vi "Registration Map Usage.vi"() -> ()   [LabVIEW 2023]
doc: "This VI demonstrates how to use the set and map data types to create a registration map with high performance."
uses:
  Do Cleaning Action.ctl
panel:
  in  "Hotel To Check":string(combo)="Four Seasons"
  in  "Stop":bool
  in  "Hotel 4":string(combo)="Four Seasons"
  in  "Unregister 4":bool
  in  "Register 4":bool
  out "Guest 4":string="Darshan"
  in  "Hotel 3":string(combo)="Four Seasons"
  in  "Unregister 3":bool
  in  "Register 3":bool
  out "Guest 3":string="Carmichael"
  in  "Hotel 2":string(combo)="Four Seasons"
  in  "Unregister 2":bool
  in  "Register 2":bool
  out "Guest 2":string="Bernice"
  in  "Hotel 1":string(combo)="Four Seasons"
  out "Event Log":string
  in  "Check":bool
  in  "Unregister 1":bool
  in  "Register 1":bool
  out "Guest 1":string="Ayita"
  # "Overview: This VI demonstrates how to use the set and map data types to create a registration map with high performance.\n\nA common requirement of software is to have one set of actors each register for some services. The services maintain the list of registered actors. Each service does setup work or starts operation only when the first actor registers and then does cleanup only after the last actor unregisters. These lookup tables often need to be quite fast despite potentially growing quite large. This example uses a set of people who are registering to stay at various hotels. When the first guest registers for a given hotel, that hotel begins a cleaning service. When the last guest unregisters from a hotel, that hotel stops its cleaning service. \n\nThe malleable VIs used in this example are resuable in any application that needs this sort of registration map, regardless of the data types of the relevant actors and services. \n\nInstructions:\n1. Run the VI.  Press buttons to register and unregister guests for various hotels. In this example, the same guest can register to stay at multiple hotels! The event log shows the latest status.\n2. Stop the VI.\n3. Open the block diagram and review further commentary there."
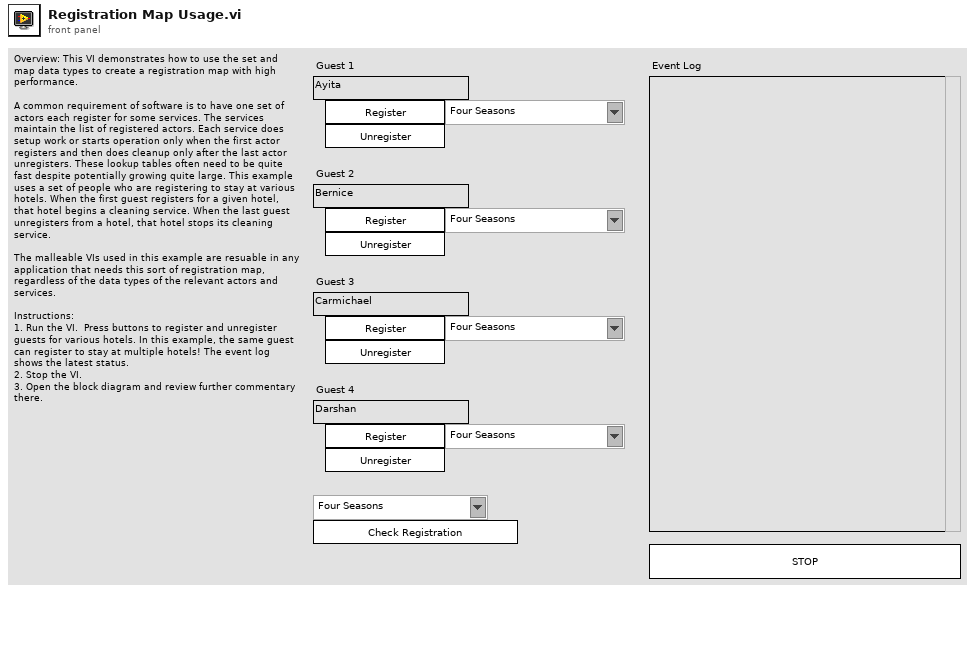
[diagram p1: front panel]
types:
  T1 = typedef "Do Cleaning Action.ctl" = enum16{"Begin", "End"}
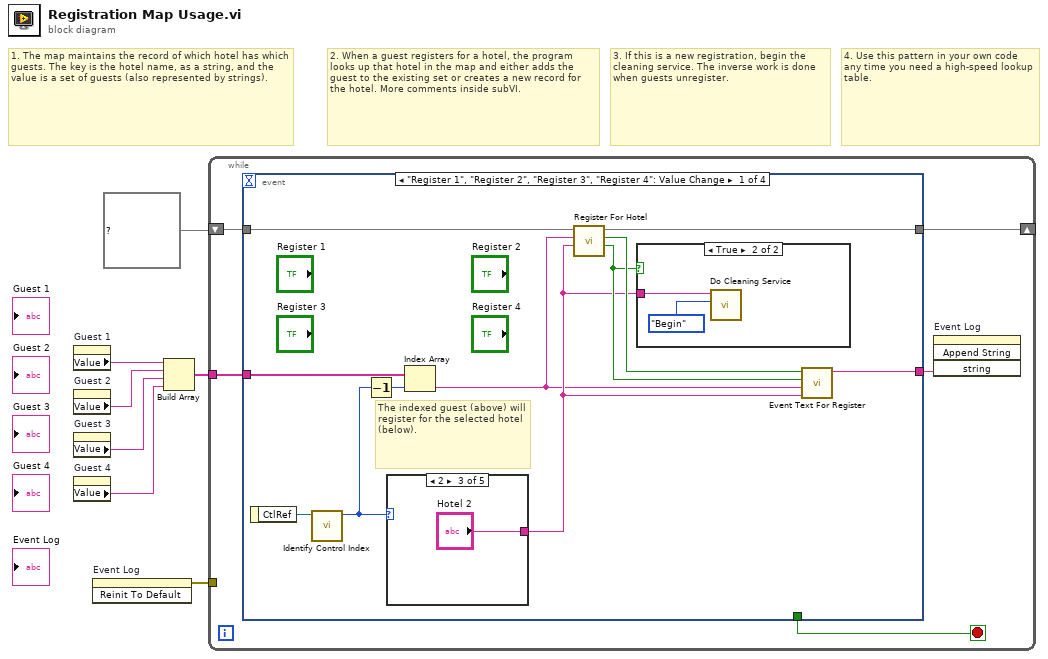
[diagram p0: block diagram]
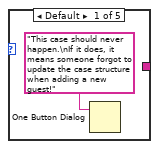
[diagram p2: hidden frame]
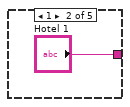
[diagram p3: hidden frame]
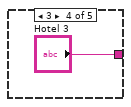
[diagram p4: hidden frame]
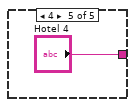
[diagram p5: hidden frame]
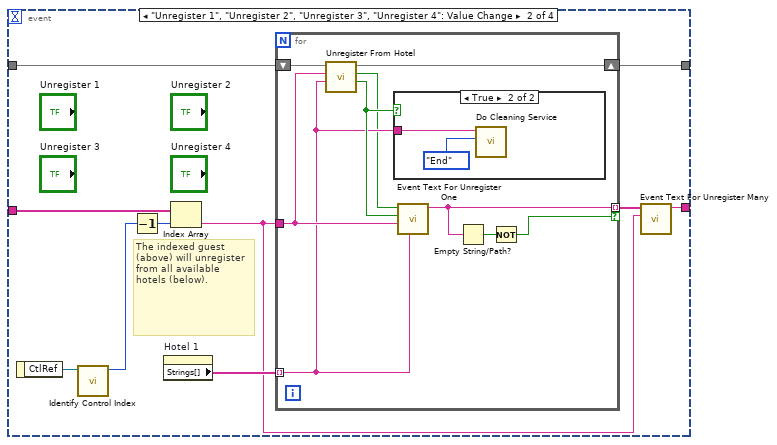
[diagram p7: hidden frame]
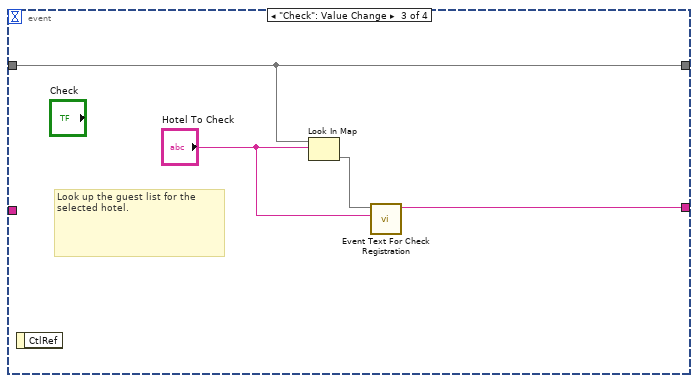
[diagram p9: hidden frame]
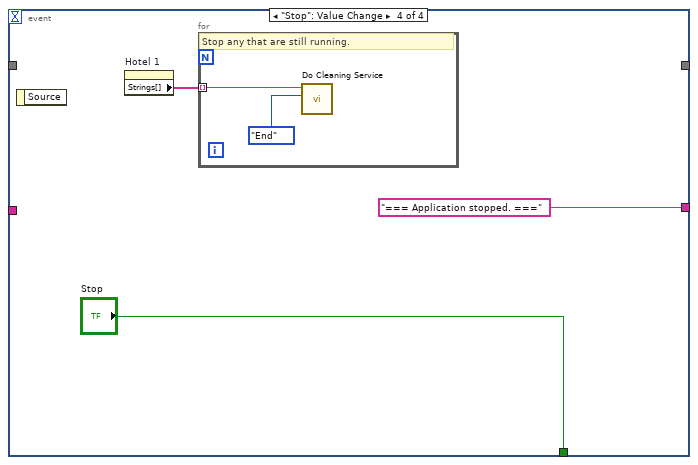
[diagram p10: hidden frame]
diagram:
  # "4. Use this pattern in your own code any time you need a high-speed lookup table."
  # "3. If this is a new registration, begin the cleaning service. The inverse work is done when guests unregister."
  # "2. When a guest registers for a hotel, the program looks up that hotel in the map and either adds the guest to the existing set or creates a new record for the hotel. More comments inside subVI."
  # "1. The map maintains the record of which hotel has which guests. The key is the hotel name, as a string, and the value is a set of guests (also represented by strings)."
  n1 = property on="Guest 1" class="Str"() -> ("Value"=w7:string)  [unwired: 2 in, 2 out]
  n2 = property on="Guest 2" class="Str"() -> ("Value"=w6:string)  [unwired: 2 in, 2 out]
  n3 = property on="Guest 3" class="Str"() -> ("Value"=w5:string)  [unwired: 2 in, 2 out]
  n4 = property on="Guest 4" class="Str"() -> ("Value"=w4:string)  [unwired: 2 in, 2 out]
  n5 = invoke on="Event Log" class="Str" method="Reinit To Default"() -> (error out=w2:errorcluster)  [unwired: 3 in, 2 out]
  n6 = Build Array(w7, w6, w5, w4) -> (w3:string[])
  n7 = while {
    tunnel: w3 -> [w11]
    shift-right: [w10] -> _
    shift-left: map{string, set{string}} {} ("map out") -> [w9]
    tunnel: w2 -> [_]
    stop <- w12 stop-if-true
    n8 = event shown="[0] \"Register 1\", \"Register 2\", \"Register 3\", \"Register 4\": Value Change" {
      selector: _ -> [_ _ _ _]
      dyn-events: _ -> [_ _ _ _]
      timeout: _ -> [_ _ _ _]
      tunnel: [_ _ _ "Stop"] -> w12
      tunnel: w11 -> [w22 w39 _ _]
      tunnel: [w14 w37 w55 _] -> w10
      tunnel: w9 -> [w15 w36 w55 _]
      tunnel: [w19 w33 w53 "=== Application stopped. ===" ("L10n_Stop message")] -> w8
      event "Register 1", "Register 2", "Register 3", "Register 4": Value Change {
        # "The indexed guest (above) will register for the selected hotel (below)."
        n9 = event-data() -> ("CtlRef"=w23:refnum<vi>)  [unwired: 1 in]
        n10 = call "Identify Control Index.vi"("control ref"=w23) -> ("index"=w21:i32)  [unwired: 10 in]
        n11 = Decrement(x=w21) -> (x-1=w18:i32)
        n12 = case shown="2" w21 {
          tunnel: [_ "Hotel 1" "Hotel 2" "Hotel 3" "Hotel 4"] -> w16
          frame Default {
            n13 = One Button Dialog(message="This case should never happen.\nIf it does, it means someone forgot to update the case structure when adding a new guest!" ("L10n_Never")) -> ()  [unwired: 1 in, 1 out]
          }
          frame 1 {
          }
          frame 2 {
          }
          frame 3 {
          }
          frame 4 {
          }
        }
        n14 = Index Array(array=w22, index=w18) -> (element=w13:string)
        n15 = call "Register For Hotel.vi"("hotel"=w16, "guest"=w13, "map in"=w15) -> ("first registration for this hotel?"=w17:bool, "guest already registered here?"=w20:bool, "map out"=w14:map{string, set{string}})  [unwired: 6 in]
        n16 = case shown="True" w17 {
          tunnel: w16 -> [_ w30]
          frame False {
          }
          frame True {
            n17 = call "Do Cleaning Service.vi"("Action"=Do_Cleaning_Action."Begin", "Hotel"=w30) -> ()  [unwired: 10 in]
          }
        }
        n18 = call "Event Text For Register.vi"("hotel"=w16, "guest"=w13, "first registration?"=w17, "already registered?"=w20) -> ("message"=w19:string)  [unwired: 7 in]
      }
      event "Unregister 1", "Unregister 2", "Unregister 3", "Unregister 4": Value Change {
        # "The indexed guest (above) will unregister from all available hotels (below)."
        n19 = event-data() -> ("CtlRef"=w40:refnum<vi>)  [unwired: 1 in]
        n20 = call "Identify Control Index.vi"("control ref"=w40) -> ("index"=w38:i32)  [unwired: 10 in]
        n21 = Decrement(x=w38) -> (x-1=w35:i32)
        n22 = property on="Hotel 1" class="CmbBox"() -> ("Strings[]"=w34:string[])  [unwired: 2 in, 2 out]
        n23 = Index Array(array=w39, index=w35) -> (element=w31:string)
        n24 = for {
          shift-right: [w49] -> w37
          shift-left: w36 -> [w48]
          tunnel: w34 -> [w45] mode=indexing
          tunnel: w31 -> [w47]
          tunnel: [w43] -> w32 mode=indexing if=w41
          n25 = call "Unregister From Hotel.vi"("hotel"=w45, "guest"=w47, "map in"=w48) -> ("removed last registration?"=w46:bool, "guest not registered for this hotel?"=w44:bool, "map out"=w49:map{string, set{string}})  [unwired: 6 in]
          n26 = case shown="True" w46 {
            tunnel: w45 -> [_ w50]
            frame False {
            }
            frame True {
              n27 = call "Do Cleaning Service.vi"("Action"=Do_Cleaning_Action."End", "Hotel"=w50) -> ()  [unwired: 10 in]
            }
          }
          n28 = call "Event Text For Unregister One.vi"("hotel"=w45, "guest"=w47, "zero registrations remaining?"=w46, "not registered?"=w44) -> ("message"=w43:string)  [unwired: 7 in]
          n29 = Empty String/Path?(string/path=w43) -> (empty?=w42:bool)
          n30 = Not(x=w42) -> (.not. x?=w41:bool)
        }
        n31 = call "Event Text For Unregister Many.vi"("guest"=w31, "strings"=w32) -> ("string"=w33:string)  [unwired: 9 in]
      }
      event "Check": Value Change {
        # "Look up the guest list for the selected hotel."
        n32 = event-data() -> ()  [unwired: 1 in, 1 out]
        n33 = Look In Map(map=w55, key="Hotel To Check") -> (value=w52:set{string})  [unwired: 1 in, 1 out]
        n34 = call "Event Text For Check Registration.vi"("hotel to check"="Hotel To Check", "guests"=w52) -> ("message"=w53:string)  [unwired: 9 in]
      }
      event "Stop": Value Change {
        n35 = event-data() -> ()  [unwired: 1 in, 1 out]
        n36 = property on="Hotel 1" class="CmbBox"() -> ("Strings[]"=w56:string[])  [unwired: 2 in, 2 out]
        n37 = for {
          tunnel: w56 -> [w60] mode=indexing
          # "Stop any that are still running."
          n38 = call "Do Cleaning Service.vi"("Action"=Do_Cleaning_Action."End", "Hotel"=w60) -> ()  [unwired: 10 in]
        }
      }
    }
    n39 = invoke on="Event Log" class="Str" method="Append String"("string"=w8) -> ()  [unwired: 3 in, 4 out]
  }
